vi "ground.vi"() -> ()   [LabVIEW 2015]
panel:
  in  "thresh":dbl=5.0 format="%#_13g"
  out "Waveform Graph 6":dbl[](graph)
  out "Waveform Graph 5":dbl[](graph)
  out "obs":i32[](array[numeric])
  in  "diff":i32=1
  out "XY Graph":cluster{"Y":dbl[], "Y":dbl[]}[](graph)
  in  "transposed array 2":dbl[][](array[numeric])
  in  "Numeric":i32=1
  out "X":dbl[](array[numeric])
  out "Y":dbl[](array[numeric])
  out "Z":dbl[](array[numeric])
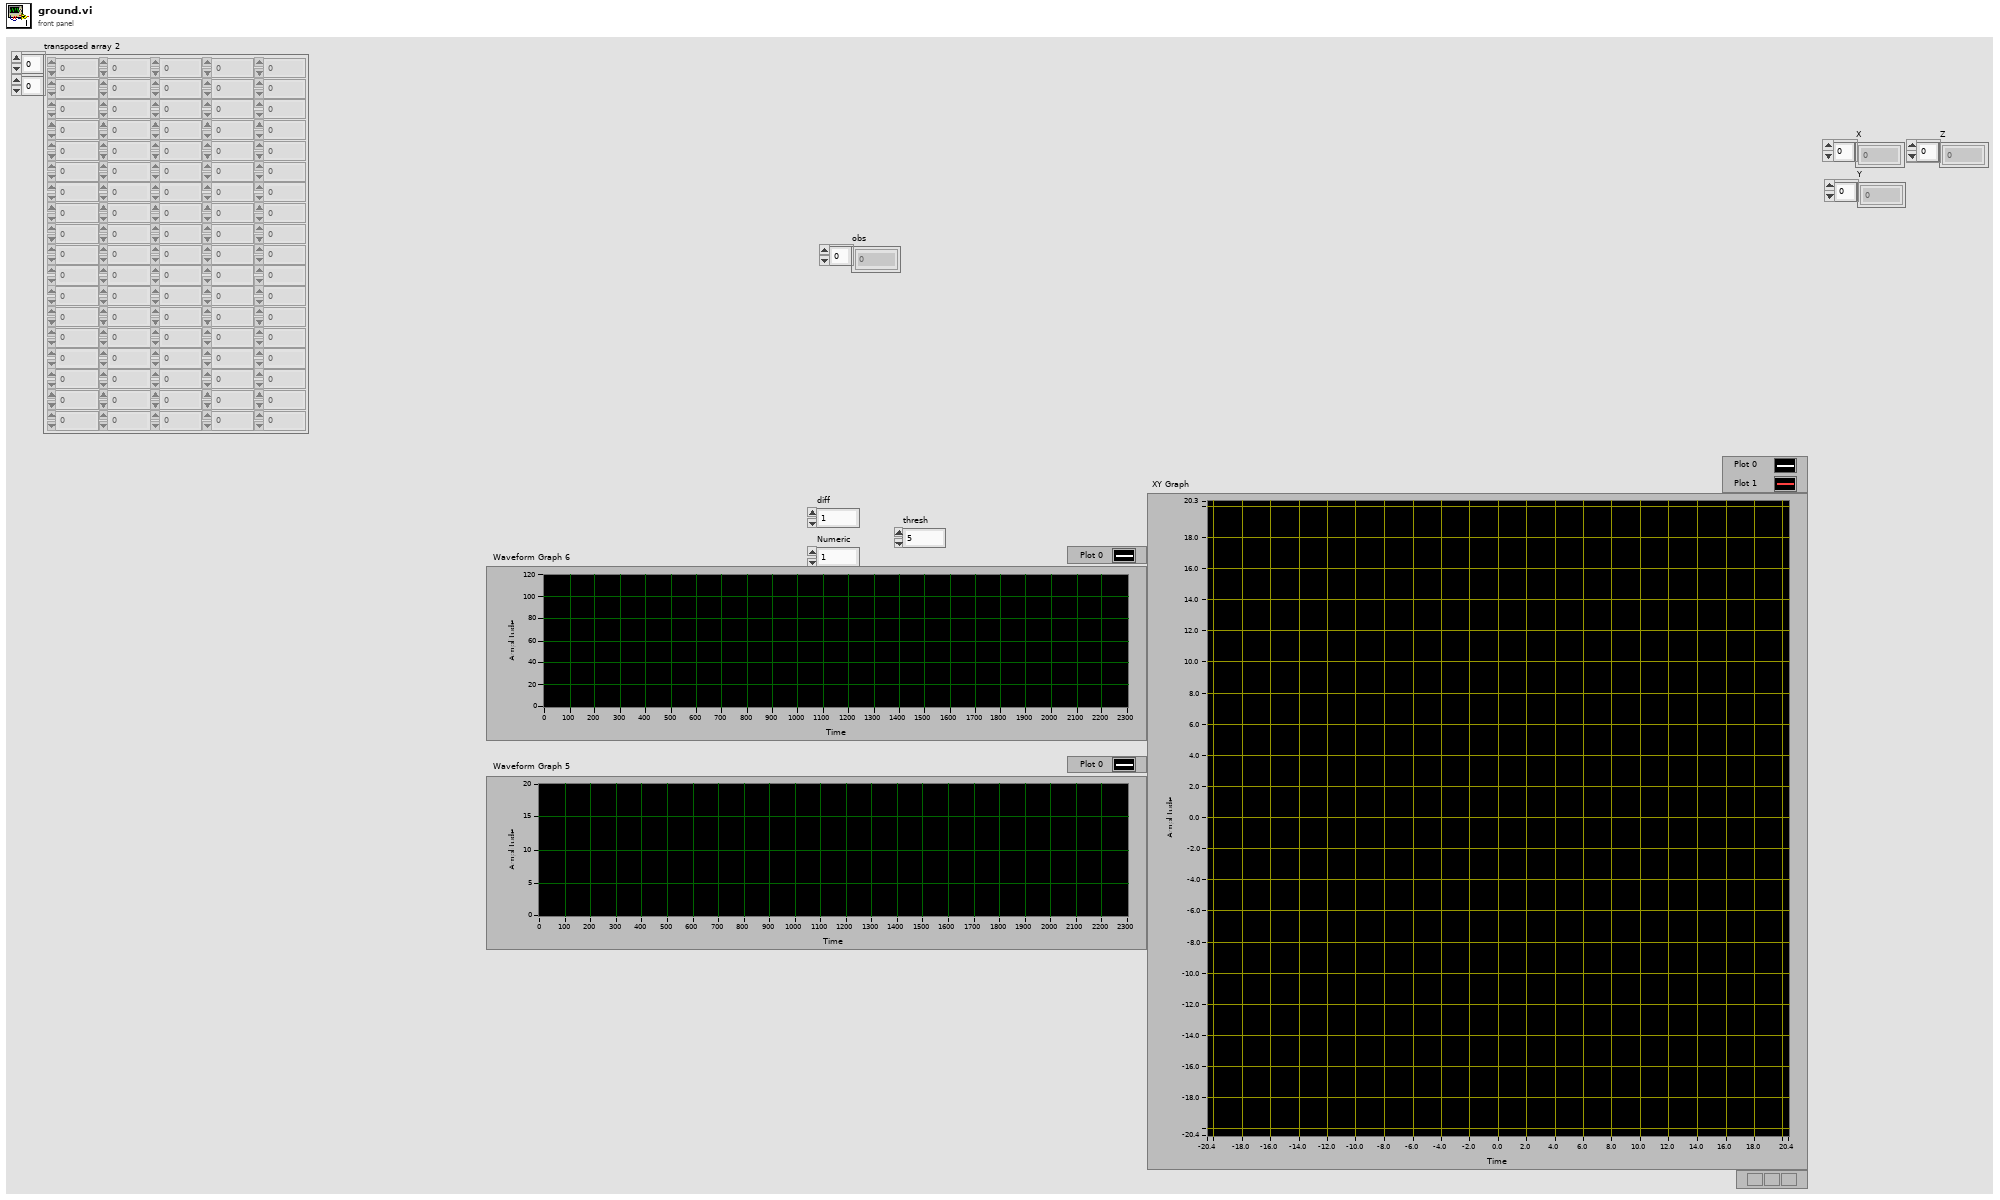
[diagram p1: front panel]
types:
  T1 = cluster{i32, "Rotational position":dbl, "Rotational position":dbl, "Rotational position":dbl}[]
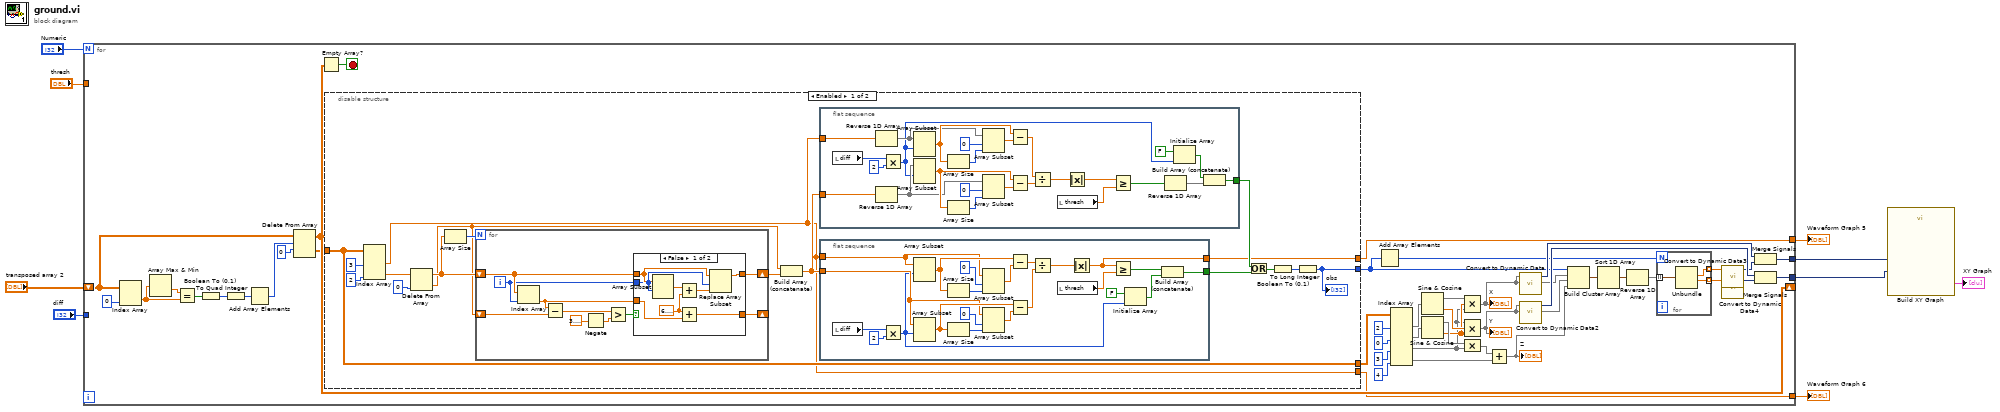
[diagram p0: block diagram]
diagram:
  n1 = for {
    N: "Numeric" -> [_]
    shift-right: [w44] -> _
    shift-left: "transposed array 2" -> [w45]
    tunnel: "diff" -> [_]
    tunnel: [w13] -> w6
    tunnel: [w12] -> w4
    tunnel: [w11] -> w3
    tunnel: [w10] -> w2
    tunnel: "thresh" -> [_]
    stop <- w32 stop-if-true
    n2 = Index Array(array=w45, index (col)=0 ("disabled index (col)")) -> (element=w51:dbl[])  [unwired: 1 in]
    n3 = Array Max & Min(array=w51) -> (min value=w52:dbl)  [unwired: 3 out]
    n4 = Equal?(x=w52, y=w51) -> (x = y?=w50:bool[])
    n5 = Boolean To (0,1)(Boolean=w50) -> (0, 1=w49:i16[])
    n6 = To Quad Integer(1:w49) -> (0:w48:i64[])
    n7 = Add Array Elements(numeric array=w48) -> (sum=w47:i64)
    n8 = Delete From Array(array=w45, length=w47, index (row)=0) -> (deleted portion=w15:dbl[][], array with subset deleted=w44:dbl[][])  [unwired: 1 in]
    n9 = Empty Array?(array=w44) -> (empty?=w32:bool)
    n10 = disable-structure shown="Enabled" {
      disable-tunnel: w15 -> [w63 _]
      disable-tunnel: [w64 _] -> w22
      disable-tunnel: [w63 _] -> w14
      disable-tunnel: [w58 _] -> w13
      disable-tunnel: [w57 _] -> w10
      frame Enabled {
        n11 = Index Array(array=w63, index (col) #1=3 ("disabled index (col)"), index (col) #2=2 ("disabled index (col)")) -> (element #1=w57:dbl[], element #2=w67:dbl[])  [unwired: 2 in]
        n12 = Delete From Array(array=w67, index=0) -> (deleted portion=w69:dbl, array with subset deleted=w71:dbl[])  [unwired: 1 in]
        n13 = Array Size(array=w71) -> (size(s)=w72:i32)
        n14 = for {
          N: w72 -> [_]
          shift-right: [w130] -> w70
          shift-left: w71 -> [w129]
          shift-right: [w128] -> _
          shift-left: w69 -> [w125]
          i -> [w127]
          n15 = Index Array(array=w129, index=w127) -> (element=w126:dbl)
          n16 = Subtract(x=w126, y=w125) -> (x-y=w122:dbl)
          n17 = Negate(x=3.141592653589793) -> (-x=w123:dbl)
          n18 = Greater?(x=w122, y=w123) -> (0:w121:bool)
          n19 = case shown="False" w121 {
            tunnel: [w134 w140] -> w130
            tunnel: w129 -> [w137 w140]
            tunnel: [w131 w139] -> w128
            tunnel: w126 -> [w132 w139]
            tunnel: w127 -> [w136 _]
            frame False {
              w133 = 6.283185307179586
              n20 = Array Subset(array=w137, index=w136) -> (w138:dbl[])  [unwired: 1 in]
              n21 = Add(x=w138, y=w133) -> (x+y=w135:dbl[])
              n22 = Add(x=w133, y=w132) -> (x+y=w131:dbl)
              n23 = Replace Array Subset(array=w137, new element=w135, index=w136) -> (w134:dbl[])
            }
            frame True {
            }
          }
        }
        n24 = Build Array (concatenate)(w69, w70) -> (w62:dbl[])
        n25 = flat-sequence {
          tunnel: w57 -> [w82]
          tunnel: w62 -> [w80]
          tunnel: [w85] -> w61
          frame #0 {
            n26 = local read "diff"() -> (w83:i32)
            n27 = Reverse 1D Array(array=w82) -> (reversed array=w81:dbl[])
            n28 = Reverse 1D Array(array=w80) -> (reversed array=w79:dbl[])
            n29 = Multiply(x=w83, y=2) -> (x*y=w75:i32)
            n30 = Array Subset(array=w81, index=w75) -> (w94:dbl[])  [unwired: 1 in]
            n31 = Array Subset(array=w79, index=w75) -> (w90:dbl[])  [unwired: 1 in]
            n32 = Array Size(array=w94) -> (size(s)=w93:i32)
            n33 = Array Size(array=w90) -> (size(s)=w89:i32)
            n34 = Array Subset(array=w81, index=0, length=w93) -> (w91:dbl[])
            n35 = Array Subset(array=w79, index=0, length=w89) -> (w87:dbl[])
            n36 = Subtract(x=w94, y=w91) -> (x-y=w97:dbl[])
            n37 = Subtract(x=w90, y=w87) -> (x-y=w98:dbl[])
            n38 = Divide(x=w97, y=w98) -> (x/y=w96:dbl[])
            n39 = local read "thresh"() -> (w74:dbl)
            n40 = Absolute Value(x=w96) -> (abs(x)=w95:dbl[])
            n41 = Greater Or Equal?(x=w95, y=w74) -> (x >= y?=w78:bool[])
            n42 = Reverse 1D Array(array=w78) -> (reversed array=w77:bool[])
            n43 = Initialize Array(FALSE, w75) -> (w76:bool[])
            n44 = Build Array (concatenate)(w76, w77) -> (w85:bool[])
          }
        }
        n45 = flat-sequence {
          tunnel: w57 -> [w116]
          tunnel: w62 -> [w110]
          tunnel: [w106] -> w60
          tunnel: [w100] -> w58
          frame #0 {
            n46 = local read "diff"() -> (w104:i32)
            n47 = Multiply(x=w104, y=2) -> (x*y=w101:i32)
            n48 = Array Subset(array=w116, index=w101) -> (w117:dbl[])  [unwired: 1 in]
            n49 = Array Subset(array=w110, index=w101) -> (w112:dbl[])  [unwired: 1 in]
            n50 = Array Size(array=w117) -> (size(s)=w115:i32)
            n51 = Array Size(array=w112) -> (size(s)=w111:i32)
            n52 = Array Subset(array=w116, index=0, length=w115) -> (w113:dbl[])
            n53 = Array Subset(array=w110, index=0, length=w111) -> (w108:dbl[])
            n54 = Subtract(x=w117, y=w113) -> (x-y=w119:dbl[])
            n55 = Subtract(x=w112, y=w108) -> (x-y=w120:dbl[])
            n56 = Divide(x=w119, y=w120) -> (x/y=w118:dbl[])
            n57 = local read "thresh"() -> (w99:dbl)
            n58 = Absolute Value(x=w118) -> (abs(x)=w100:dbl[])
            n59 = Greater Or Equal?(x=w100, y=w99) -> (x >= y?=w102:bool[])
            n60 = Initialize Array(FALSE, w101) -> (w103:bool[])
            n61 = Build Array (concatenate)(w102, w103) -> (w106:bool[])
          }
        }
        n62 = Or(x=w61, y=w60) -> (x .or. y?=w59:bool[])
        n63 = Boolean To (0,1)(Boolean=w59) -> (0, 1=w65:i16[])
        n64 = To Long Integer(number=w65) -> (32bit integer=w64:i32[])
        "obs" <- w64
      }
      frame Disabled {
      }
    }
    n65 = Add Array Elements(numeric array=w22) -> (sum=w21:i32)
    n66 = Index Array(array=w14, index (col) #1=2 ("disabled index (col)"), index (col) #2=0 ("index (col)"), index (col) #3=3 ("index (col)"), index (col) #4=4 ("index (col)")) -> (element #1=w31:dbl[], element #2=w36:dbl[], element #3=w30:dbl[], element #4=w33:dbl[])  [unwired: 4 in]
    n67 = Sine & Cosine(0:w31) -> (1:w40:dbl[], 2:w41:dbl[])
    n68 = Sine & Cosine(0:w36) -> (1:w42:dbl[], 2:w39:dbl[])
    n69 = Compound Arithmetic op=MULTIPLY(w40, w39, w30) -> (w27:dbl[])
    "X" <- w27
    n70 = Compound Arithmetic op=MULTIPLY(w30, w41, w39) -> (w26:dbl[])
    "Y" <- w26
    n71 = Compound Arithmetic op=MULTIPLY(w42, w30) -> (w43:dbl[])
    n72 = Add(x=w43, y=w33) -> (x+y=w25:dbl[])
    "Z" <- w25
    n73 = call "Convert to Dynamic Data"("Array"=w27) -> ("Dynamic Data Type"=w29:dynamicdata)  [unwired: 3 in]
    n74 = call "Convert to Dynamic Data2"("Array"=w26) -> ("Dynamic Data Type"=w28:dynamicdata)  [unwired: 3 in]
    n75 = Build Cluster Array(w22, w27, w26, w25) -> (w24:T1)
    n76 = Sort 1D Array(array=w24) -> (sorted array=w23:T1)
    n77 = Reverse 1D Array(array=w23) -> (reversed array=w20:T1)
    n78 = for {
      N: w21 -> [_]
      tunnel: w20 -> [w56] mode=indexing
      tunnel: [w55] -> w19 mode=indexing
      tunnel: [w54] -> w17 mode=indexing
      n79 = Unbundle(w56) -> ("Rotational position"=w55:dbl, "Rotational position"=w54:dbl)  [unwired: 2 out]
    }
    n80 = call "Convert to Dynamic Data3"("Array"=w19) -> ("Dynamic Data Type"=w18:dynamicdata)  [unwired: 3 in]
    n81 = call "Convert to Dynamic Data4"("Array"=w17) -> ("Dynamic Data Type"=w16:dynamicdata)  [unwired: 3 in]
    n82 = Merge Signals(w29, w18) -> (w12:dynamicdata)
    n83 = Merge Signals(w28, w16) -> (w11:dynamicdata)
  }
  "Waveform Graph 5" <- w6
  "Waveform Graph 6" <- w2
  n84 = call "Build XY Graph"("Y Input"=w3, "X Input"=w4) -> ("XY Graph"=→"XY Graph":cluster{"X":dbl[], "Y":dbl[]}[])  [unwired: 8 in, 1 out]
